vi "Mouse Down_ on Plot.vi"(7 "PlatMods":T1, 8 "error in (no error)":errorcluster, 10 "Y axes":refnum<vi>[](array[refnum]), 11 "Meta LUT":refnum<data-value>) -> (0 "error out":errorcluster, 2 "scale index":i32[](array[numeric]), 3 "axes to scale":refnum<vi>[](array[refnum]))   [LabVIEW 2021, in "RocketPlot.lvlib"]
uses:
  RocketPlot.lvlib
  Plot scale refnum to LUT name.vi
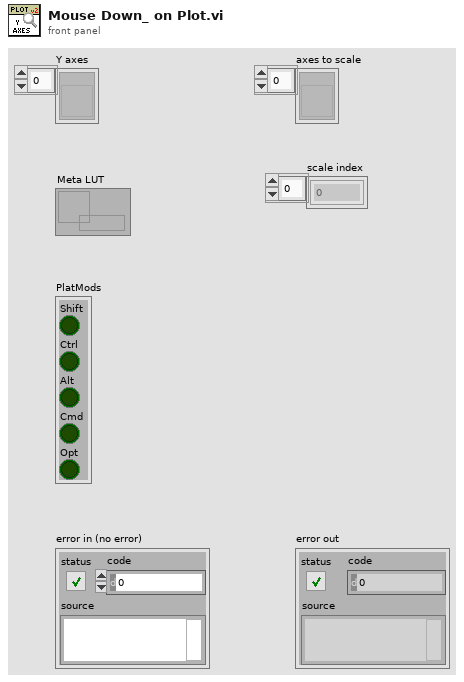
[diagram p1: front panel]
types:
  T1 = cluster{"Shift":bool, "Ctrl":bool, "Alt":bool, "Cmd":bool, "Opt":bool}
  T2 = typedef "RocketPlot.lvlib/Plot scale meta JSON.ctl" = cluster{"Type":T3, "Grid Colors:Major Color":u32, "Grid Colors:Minor Color":u32, "Style":u8, "Tick Colors:Tick Color":u32, "Tick Colors:Minor Tick Color":u32, "Format String":string, "State":T4, "AxisFocus":refnum<vi>}
  T3 = typedef "RocketPlot.lvlib/Plot axis.ctl" = enum16{"x axis", "left axis", "right axis"}
  T4 = typedef "RocketPlot.lvlib/Plot scale meta state.ctl" = cluster{"Visible":bool, "Focus":bool, "Multi-Y":bool}
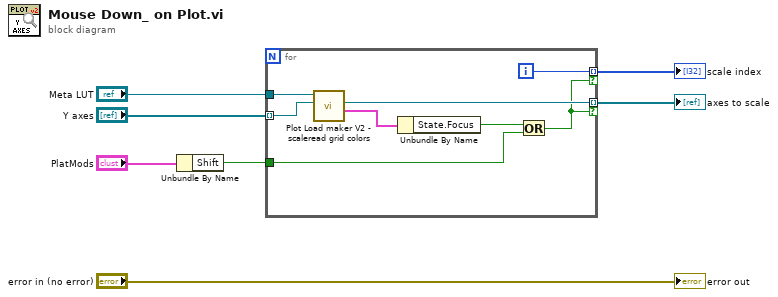
[diagram p0: block diagram]
diagram:
  n1 = Unbundle By Name("PlatMods") -> ("Shift"=w6:bool)
  n2 = for {
    tunnel: "Meta LUT" -> [w15]
    tunnel: "Y axes" -> [w13] mode=indexing
    tunnel: w6 -> [w11]
    tunnel: [w10] -> w2 mode=indexing if=w8
    tunnel: [w9] -> w1 mode=indexing if=w8
    i -> [w9]
    n3 = call "Plot Load maker V2 - scaleread grid colors.vi"("Scale reference"=w13, "Meta LUT"=w15) -> ("Scale LUT meta"=w14:T2, "Scale reference"=w10:refnum<vi>)  [unwired: 6 in, 2 out]
    n4 = Unbundle By Name(w14) -> ("State.Focus"=w12:bool)
    n5 = Or(x=w12, y=w11) -> (x .or. y?=w8:bool)
  }
  "axes to scale" <- w2
  "scale index" <- w1
  "error out" <- "error in (no error)"
